vi "Disconnect.vi"(8 "error in":errorcluster, 11 "SL_SC in":refnum<class "SL_SC.lvclass">) -> (0 "error out":errorcluster, 3 "SL_SC out":refnum<class "SL_SC.lvclass">)   [LabVIEW 2019, in "SL_SC.lvlib" / "SL_SC.lvclass"]
doc: "This override VI is a carryover override from the parent class, children classes *must* override this VI and therefore the parent class must contain this VI to maintain the override rules."
uses:
  Library/SL_SC.lvclass
  Library/SL_SC.lvclass/SL_SC.ctl
  <vilib>/SLSC/Close Session.vi
  builds/Instruments/DIG_IO.lvlibp/Library/DIG_IO.lvclass
  <vilib>/SLSC/SLSC.lvlib
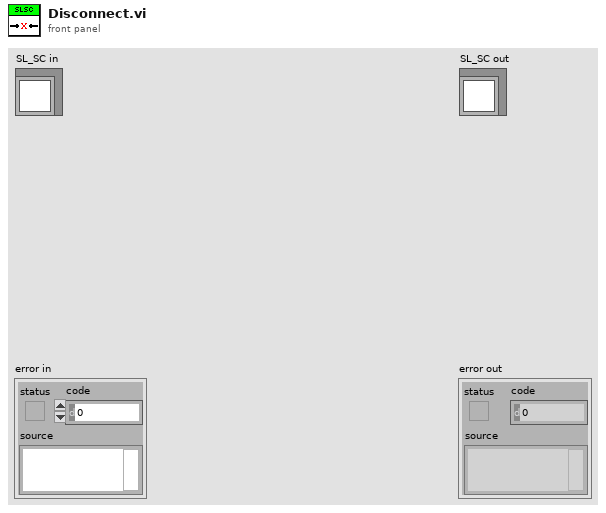
[diagram p1: front panel]
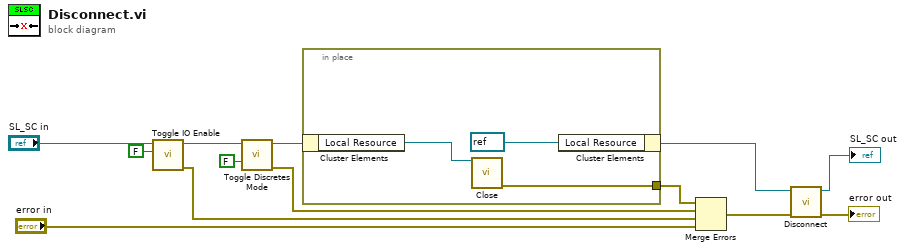
[diagram p0: block diagram]
diagram:
  n1 = call-dynamic "Toggle IO Enable.vi"("IO_EN"=FALSE, "SL_SC in"="SL_SC in") -> ("error out"=w3:errorcluster, "SL_SC out"=w4:refnum<class "SL_SC.lvclass">)  [unwired: 8 in]
  n2 = call "Toggle Discretes Mode.vi"("Discrete_Enable"=FALSE, "SL_SC in"=w4) -> ("error out"=w6:errorcluster, "SL_SC out"=w9:refnum<class "SL_SC.lvclass">)  [unwired: 8 in]
  n3 = in-place {
    in-place-border: [w16] -> w7
    n4 = in-place-cluster #1(w9) -> ("Local Resource"=w15:refnum<k21>)
    n5 = call-poly <vilib>:"Close.vi"("session in"=w15) -> ("error out"=w16:errorcluster)  [unwired: 14 in]
    n6 = in-place-cluster #1("Local Resource"=refnum<k21> refnum) -> (w11:refnum<class "SL_SC.lvclass">)
  }
  n7 = Merge Errors(w7, w6, w3, "error in") -> (w10:errorcluster)
  n8 = call-parent "Disconnect.vi"("error in"=w10, "DIG_IO in"=w11) -> ("error out"=→"error out":errorcluster, "DIG_IO out"=→"SL_SC out":refnum<class "SL_SC.lvclass">)  [unwired: 8 in]
